vi "Set XML Path.vi"(8 "error in (no error)":errorcluster, 10 "XML Path":path, 11 "RIO Target in":refnum<class "RIO Target.lvclass">) -> (0 "error out":errorcluster, 3 "RIO Target out":refnum<class "RIO Target.lvclass">)   [LabVIEW 2014, in "RIO Target.lvclass"]
uses:
  RIO Target.lvclass
  RIO Target Configuration/RIO Target Configuration.lvclass
  RIO Target.lvclass/RIO Target.ctl
  RIO Target Configuration/RIO Target Configuration.lvclass/RIO Target Configuration.ctl
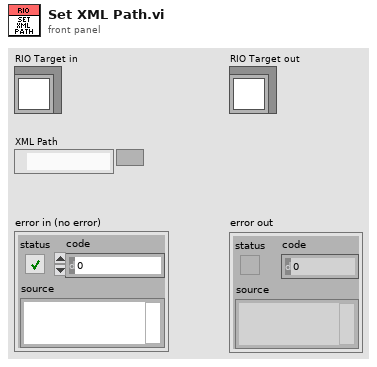
[diagram p1: front panel]
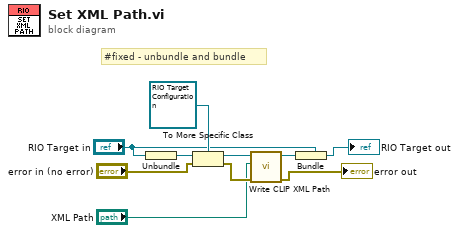
[diagram p0: block diagram]
diagram:
  # "#fixed - unbundle and bundle"
  n1 = Unbundle("RIO Target in") -> (w6:refnum<class "RIO Target Configuration.lvclass">)
  n2 = To More Specific Class(target class=refnum<class "RIO Target Configuration.lvclass"> refnum ("RIO Target Configuration in"), reference=w6, error in="error in (no error)") -> (specific class reference=w9:refnum<class "RIO Target Configuration.lvclass">, error out=w10:errorcluster)
  n3 = call "Write CLIP XML Path.vi"("error in (no error)"=w10, "CLIP XML Path"="XML Path", "RIO Target Configuration in"=w9) -> ("error out"=→"error out":errorcluster, "RIO Target Configuration out"=w4:refnum<class "RIO Target Configuration.lvclass">)  [unwired: 7 in]
  n4 = Bundle(cluster="RIO Target in", w4) -> (→"RIO Target out":refnum<class "RIO Target.lvclass">)
